vi "Get Port Widths in Bits.vi"(11 "niInstr AXI4-Stream Writer v1 FPGA in":refnum<class "niInstr AXI4-Stream Writer v1 FPGA.lvclass">) -> (2 "port widths":T1, 3 "niInstr AXI4-Stream Writer v1 FPGA out":refnum<class "niInstr AXI4-Stream Writer v1 FPGA.lvclass">)   [LabVIEW 2015, in "niInstr AXI4-Stream Writer v1 FPGA.lvclass"]
uses:
  <instrlib>/_niInstr/CLIP Adapters/v1/FPGA/AXI4-Stream/Writer/niInstr AXI4-Stream Writer v1 FPGA.lvclass
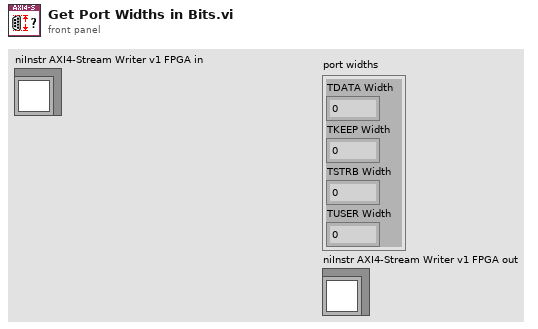
[diagram p1: front panel]
types:
  T1 = cluster{"TDATA Width":i16, "TKEEP Width":i16, "TSTRB Width":i16, "TUSER Width":i16}
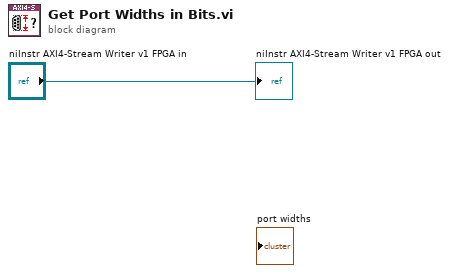
[diagram p0: block diagram]
diagram:
  "niInstr AXI4-Stream Writer v1 FPGA out" <- "niInstr AXI4-Stream Writer v1 FPGA in"
